vi "新剖面数据组合.vi"(10 "columns":string[](array[string]), 11 "剖面数据":string[][](array[string])) -> (3 "结果字符串":string)   [LabVIEW 2016, in "数据传输系统.lvlib"]
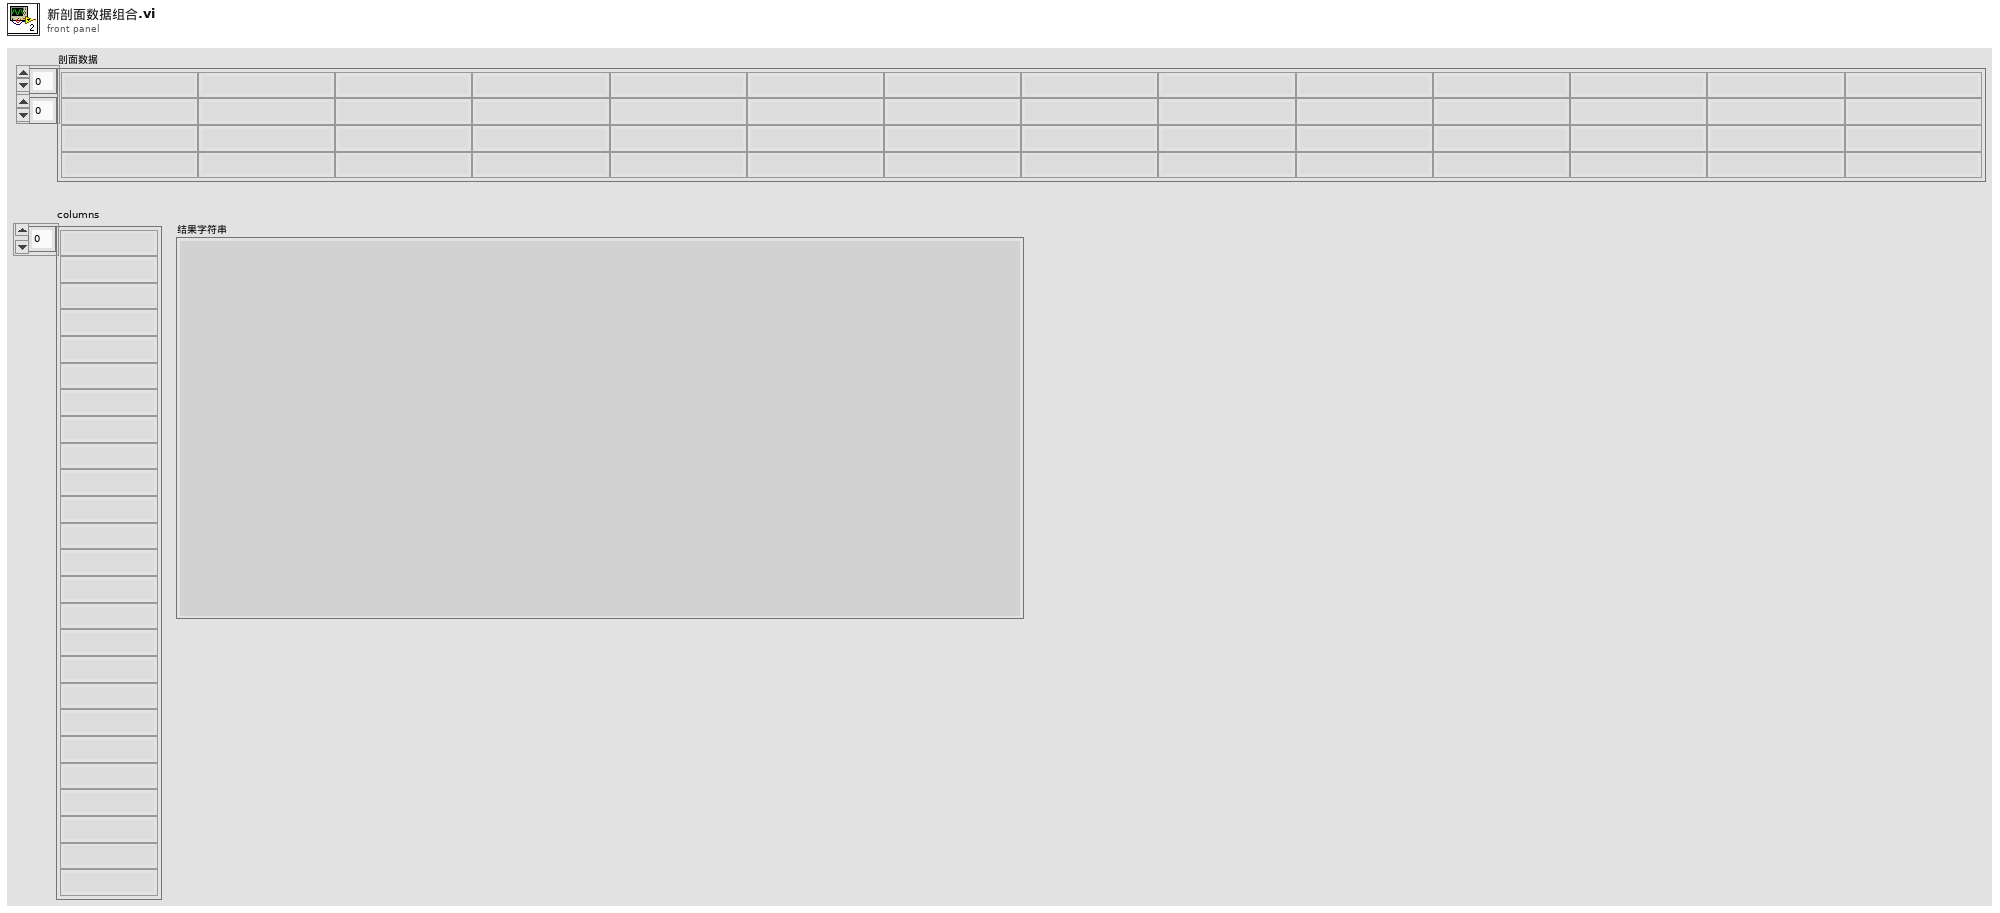
[diagram p1: front panel]
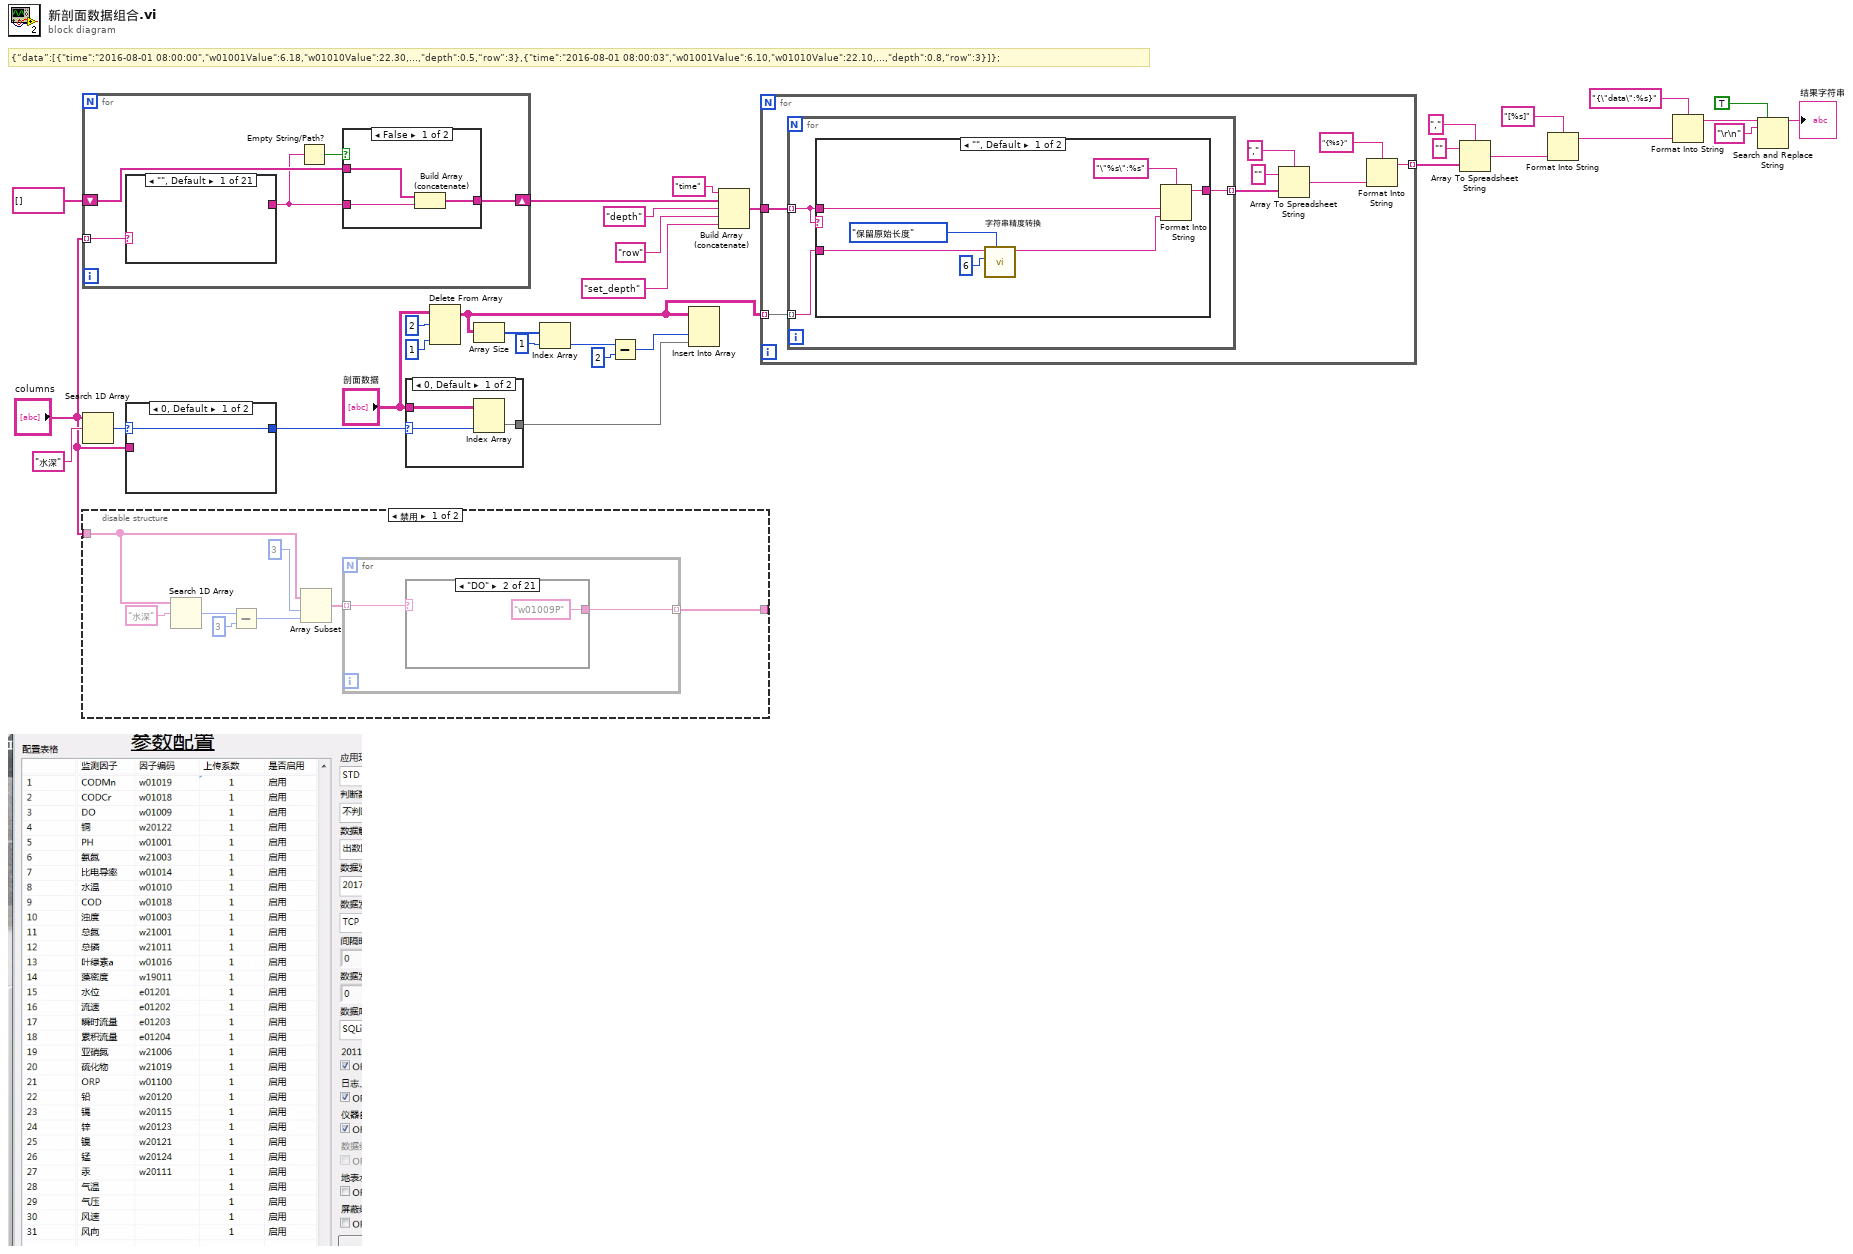
[diagram p0: block diagram]
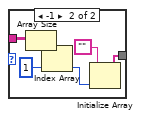
[diagram p2: hidden frame]
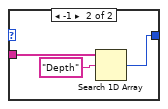
[diagram p3: hidden frame]
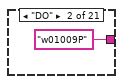
[diagram p5: hidden frame]
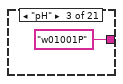
[diagram p6: hidden frame]
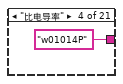
[diagram p7: hidden frame]
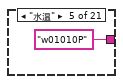
[diagram p8: hidden frame]
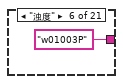
[diagram p9: hidden frame]
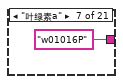
[diagram p10: hidden frame]
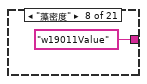
[diagram p11: hidden frame]
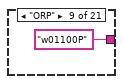
[diagram p12: hidden frame]
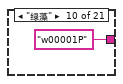
[diagram p13: hidden frame]
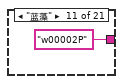
[diagram p14: hidden frame]
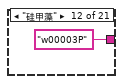
[diagram p15: hidden frame]
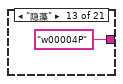
[diagram p16: hidden frame]
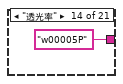
[diagram p17: hidden frame]
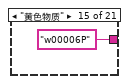
[diagram p18: hidden frame]
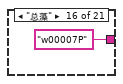
[diagram p19: hidden frame]
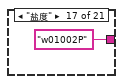
[diagram p20: hidden frame]
diagram:
  # "{“data”:[{\"time\":\"2016-08-01 08:00:00\",\"w01001Value\":6.18,\"w01010Value\":22.30,…,\"depth\":0.5,“row”:3},{\"time\":\"2016-08-01 08:00:03\",\"w01001Value\":6.10,\"w01010Value\":22.10,…,\"depth\":0.8,“row”:3}]};"
  n1 = for {
    tunnel: "columns" -> [w37] mode=indexing
    shift-right: [w34] -> w13
    shift-left: string[] [] -> [w35]
    n2 = case shown="\"\", Default" w37 {
      tunnel: [_ "w01009P" "w01001P" "w01014P" "w01010P" "w01003P" "w01016P" "w19011Value" "w01100P" "w00001P" "w00002P" "w00003P" "w00004P" "w00005P" "w00006P" "w00007P" "w01002P" "w01022P" "w81024P" "w81025P" "w81023P"] -> w33
      frame "", Default {
      }
      frame "DO" {
      }
      frame "pH" {
      }
      frame "比电导率" {
      }
      frame "水温" {
      }
      frame "浊度" {
      }
      frame "叶绿素a" {
      }
      frame "藻密度" {
      }
      frame "ORP" {
      }
      frame "绿藻" {
      }
      frame "蓝藻" {
      }
      frame "硅甲藻" {
      }
      frame "隐藻" {
      }
      frame "透光率" {
      }
      frame "黄色物质" {
      }
      frame "总藻" {
      }
      frame "盐度" {
      }
      frame "蓝绿藻" {
      }
      frame "Fv/Fm" {
      }
      frame "PAR" {
      }
      frame "GPP" {
      }
    }
    n3 = Empty String/Path?(string/path=w33) -> (empty?=w36:bool)
    n4 = case shown="False" w36 {
      tunnel: w35 -> [w40 w41]
      tunnel: [w38 w41] -> w34
      tunnel: w33 -> [w39 _]
      frame False {
        n5 = Build Array (concatenate)(w40, w39) -> (w38:string[])
      }
      frame True {
      }
    }
  }
  n6 = Search 1D Array(1D array="columns", element="水深" ("元素")) -> (index of element=w11:i32)  [unwired: 1 in]
  n7 = disable-structure shown="禁用" {
    disable-tunnel: [w64 _] -> _
    disable-tunnel: "columns" -> [w62 _]
    frame Disabled {
      n8 = Search 1D Array(1D array=w62, element="水深" ("元素")) -> (index of element=w63:i32)  [unwired: 1 in]
      n9 = Subtract(x=w63, y=3) -> (x-y=w65:i32)
      n10 = Array Subset(array=w62, index=3 ("索引"), length=w65) -> (w66:string[])
      n11 = for {
        tunnel: w66 -> [w71] mode=indexing
        tunnel: [w70] -> w64 mode=indexing
        n12 = case shown="\"DO\"" w71 {
          tunnel: [_ "w01009P" "w01001P" "w01014P" "w01010P" "w01003P" "w01016P" "w19011Value" "w01100P" "w00001P" "w00002P" "w00003P" "w00004P" "w00005P" "w00006P" "w00007P" "w01002P" "w01022P" "w81024P" "w81025P" "w81023P"] -> w70
          frame "", Default {
          }
          frame "DO" {
          }
          frame "pH" {
          }
          frame "比电导率" {
          }
          frame "水温" {
          }
          frame "浊度" {
          }
          frame "叶绿素a" {
          }
          frame "藻密度" {
          }
          frame "ORP" {
          }
          frame "绿藻" {
          }
          frame "蓝藻" {
          }
          frame "硅甲藻" {
          }
          frame "隐藻" {
          }
          frame "透光率" {
          }
          frame "黄色物质" {
          }
          frame "总藻" {
          }
          frame "盐度" {
          }
          frame "蓝绿藻" {
          }
          frame "Fv/Fm" {
          }
          frame "PAR" {
          }
          frame "GPP" {
          }
        }
      }
    }
    frame Enabled {
    }
  }
  n13 = case shown="0, Default" w11 {
    selector: w11 -> [w92 _]
    tunnel: [w92 w94] -> w10
    tunnel: "columns" -> [_ w93]
    frame 0, Default {
    }
    frame -1 {
      n14 = Search 1D Array(1D array=w93, element="Depth" ("元素")) -> (index of element=w94:i32)  [unwired: 1 in]
    }
  }
  n15 = case shown="0, Default" w10 {
    selector: w10 -> [w97 _]
    tunnel: [w96 w99] -> w4
    tunnel: "剖面数据" -> [w98 w104]
    frame 0, Default {
      n16 = Index Array(array=w98, index (col)=w97) -> (element=w96:string[])  [unwired: 1 in]
    }
    frame -1 {
      n17 = Array Size(array=w104) -> (size(s)=w103:i32[])
      n18 = Index Array(array=w103, index=1 ("索引")) -> (element=w101:i32)
      n19 = Initialize Array("", w101) -> (w99:string[])
    }
  }
  n20 = Delete From Array(array="剖面数据", length=2 ("长度"), index (col)=1 ("禁用的索引 (列)")) -> (array with subset deleted=w1:string[][])  [unwired: 1 in, 1 out]
  n21 = Array Size(array=w1) -> (size(s)=w9:i32[])
  n22 = Index Array(array=w9, index=1 ("索引")) -> (element=w7:i32)
  n23 = Subtract(x=w7, y=2) -> (x-y=w5:i32)
  n24 = Insert Into Array(array=w1, index (col)=w5, new element=w4) -> ()  [unwired: 1 in, 1 out]
  n25 = Build Array (concatenate)("time" ("元素"), w13, "depth" ("元素"), "row" ("元素"), "set_depth" ("元素")) -> (w31:string[])
  n26 = for {
    tunnel: w1 -> [w111] mode=indexing
    tunnel: w31 -> [w112]
    tunnel: [w106] -> w26 mode=indexing
    n27 = for {
      tunnel: w112 -> [w114] mode=indexing
      tunnel: w111 -> [w113] mode=indexing
      tunnel: [w115] -> w108 mode=indexing
      n28 = case shown="\"\", Default" w114 {
        tunnel: [w121 w129] -> w115
        tunnel: w114 -> [w120 w128]
        tunnel: w113 -> [w119 w124]
        frame "", Default {
          n29 = call "字符串精度转换.vi"("枚举"=enum16{"小数位修约", "保留原始长度"}."保留原始长度", "数据精度"=6, "输入字符串"=w119) -> ("输出字符串"=w116:string)  [unwired: 7 in, 1 out]
          n30 = Format Into String(format string="\"%s\":%s" ("格式字符串"), w120, w116) -> (resulting string=w121:string)  [unwired: 2 in, 1 out]
        }
        frame "time" {
          n31 = Search and Replace String(replace all?=TRUE ("替换全部？(F)"), input string=w124, search string="/" ("搜索字符串"), replace string="-" ("替换字符串(\"\")")) -> (result string=w123:string)  [unwired: 4 in, 3 out]
          n32 = Format Into String(format string="\"%s\":\"%s\"" ("格式字符串"), w128, w123) -> (resulting string=w129:string)  [unwired: 2 in, 1 out]
        }
      }
    }
    n33 = Array To Spreadsheet String(delimiter (Tab)="," ("分隔符(Tab)"), array=w108, 3:"" ("格式字符串")) -> (spreadsheet string=w105:string)
    n34 = Format Into String(format string="{%s}" ("格式字符串"), w105) -> (resulting string=w106:string)  [unwired: 2 in, 1 out]
  }
  n35 = Array To Spreadsheet String(delimiter (Tab)="," ("分隔符(Tab)"), array=w26, 3:"" ("格式字符串")) -> (spreadsheet string=w22:string)
  n36 = Format Into String(format string="[%s]" ("格式字符串"), w22) -> (resulting string=w23:string)  [unwired: 2 in, 1 out]
  n37 = Format Into String(format string="{\"data\":%s}" ("格式字符串"), w23) -> (resulting string=w19:string)  [unwired: 2 in, 1 out]
  n38 = Search and Replace String(replace all?=TRUE ("替换全部？(F)"), input string=w19, search string="\r\n") -> (result string=→"结果字符串":string)  [unwired: 5 in, 3 out]
